vi "XBox-Init.vi"(11 "error in (no error)":errorcluster) -> (4 "XBox Events":T2, 14 "Events Ref":T1, 15 "error out":errorcluster)   [LabVIEW 2015]
uses:
  XBox-Button Event.ctl
  XBox-Events Ref.ctl
  XBox-Globals.vi
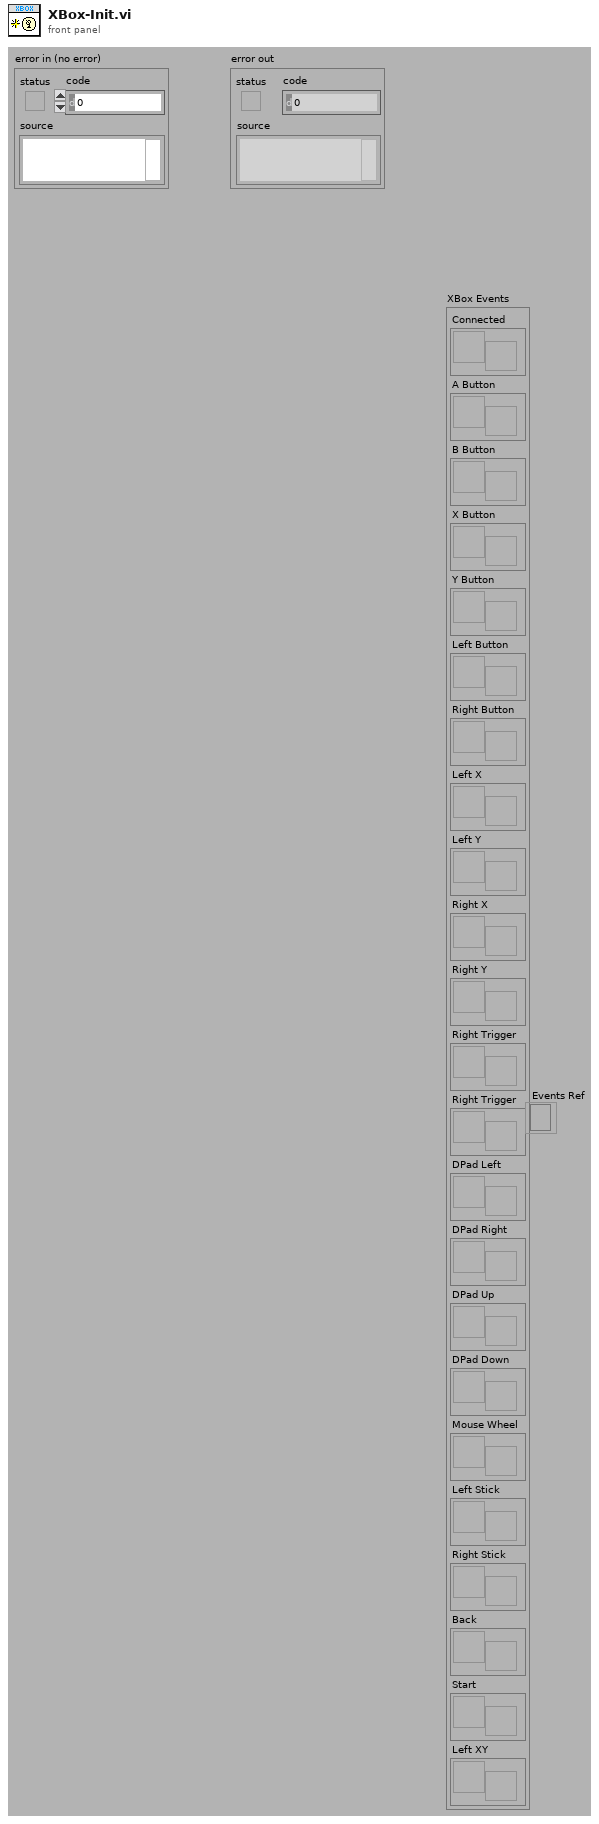
[diagram p1: front panel]
types:
  T1 = typedef "XBox-Events Ref.ctl" = refnum<event-registration>
  T2 = cluster{"Connected":refnum<user-event>, "A Button":refnum<user-event>, "B Button":refnum<user-event>, "X Button":refnum<user-event>, "Y Button":refnum<user-event>, "Left Button":refnum<user-event>, "Right Button":refnum<user-event>, "Left X":refnum<user-event>, "Left Y":refnum<user-event>, "Right X":refnum<user-event>, "Right Y":refnum<user-event>, "Right Trigger":refnum<user-event>, "Right Trigger":refnum<user-event>, "DPad Left":refnum<user-event>, "DPad Right":refnum<user-event>, "DPad Up":refnum<user-event>, "DPad Down":refnum<user-event>, "Mouse Wheel":refnum<user-event>, "Left Stick":refnum<user-event>, "Right Stick":refnum<user-event>, "Back":refnum<user-event>, "Start":refnum<user-event>, "Left XY":refnum<user-event>}
  T3 = typedef "XBox-Button Event.ctl" = cluster{"Down":bool, "Pressed":bool, "Released":bool}
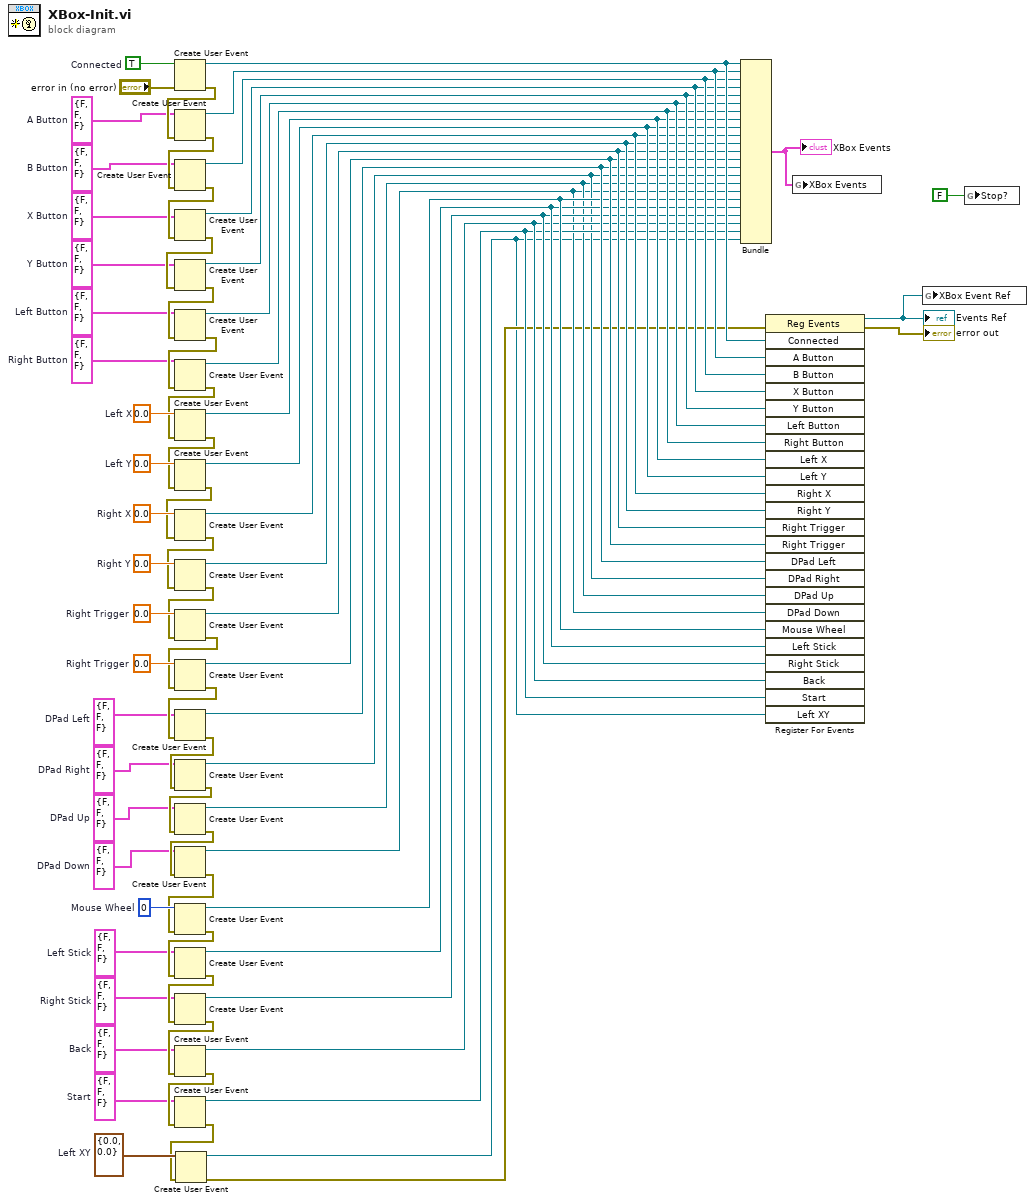
[diagram p0: block diagram]
diagram:
  w5 = cluster{"X":dbl, "Y":dbl} {"X"=0.0, "Y"=0.0}  # Left XY
  w10 = T3 {"Down"=FALSE, "Pressed"=FALSE, "Released"=FALSE}  # DPad Down
  w11 = T3 {"Down"=FALSE, "Pressed"=FALSE, "Released"=FALSE}  # DPad Up
  w12 = T3 {"Down"=FALSE, "Pressed"=FALSE, "Released"=FALSE}  # DPad Right
  w13 = T3 {"Down"=FALSE, "Pressed"=FALSE, "Released"=FALSE}  # DPad Left
  w18 = T3 {"Down"=FALSE, "Pressed"=FALSE, "Released"=FALSE}  # Start
  w19 = T3 {"Down"=FALSE, "Pressed"=FALSE, "Released"=FALSE}  # Back
  w20 = T3 {"Down"=FALSE, "Pressed"=FALSE, "Released"=FALSE}  # Right Stick
  w21 = T3 {"Down"=FALSE, "Pressed"=FALSE, "Released"=FALSE}  # Left Stick
  w22 = T3 {"Down"=FALSE, "Pressed"=FALSE, "Released"=FALSE}  # Right Button
  w23 = T3 {"Down"=FALSE, "Pressed"=FALSE, "Released"=FALSE}  # Left Button
  w24 = T3 {"Down"=FALSE, "Pressed"=FALSE, "Released"=FALSE}  # Y Button
  w25 = T3 {"Down"=FALSE, "Pressed"=FALSE, "Released"=FALSE}  # X Button
  w26 = T3 {"Down"=FALSE, "Pressed"=FALSE, "Released"=FALSE}  # B Button
  w27 = T3 {"Down"=FALSE, "Pressed"=FALSE, "Released"=FALSE}  # A Button
  w67 = TRUE  # Connected
  w68 = 0  # Mouse Wheel
  w69 = 0.0  # Right Trigger
  w70 = 0.0  # Right Trigger
  w71 = 0.0  # Right Y
  w72 = 0.0  # Right X
  w73 = 0.0  # Left Y
  w74 = 0.0  # Left X
  n1 = Create User Event(user event datatype=w67, error in="error in (no error)") -> (user event=w51:refnum<user-event>, error out=w66:errorcluster)
  n2 = Create User Event(user event datatype=w27, error in=w66) -> (user event=w50:refnum<user-event>, error out=w65:errorcluster)
  n3 = Create User Event(user event datatype=w26, error in=w65) -> (user event=w49:refnum<user-event>, error out=w64:errorcluster)
  n4 = Create User Event(user event datatype=w25, error in=w64) -> (user event=w48:refnum<user-event>, error out=w63:errorcluster)
  n5 = Create User Event(user event datatype=w24, error in=w63) -> (user event=w47:refnum<user-event>, error out=w62:errorcluster)
  n6 = Create User Event(user event datatype=w23, error in=w62) -> (user event=w46:refnum<user-event>, error out=w61:errorcluster)
  n7 = Create User Event(user event datatype=w22, error in=w61) -> (user event=w45:refnum<user-event>, error out=w60:errorcluster)
  n8 = Create User Event(user event datatype=w74, error in=w60) -> (user event=w44:refnum<user-event>, error out=w59:errorcluster)
  n9 = Create User Event(user event datatype=w73, error in=w59) -> (user event=w43:refnum<user-event>, error out=w58:errorcluster)
  n10 = Create User Event(user event datatype=w72, error in=w58) -> (user event=w42:refnum<user-event>, error out=w57:errorcluster)
  n11 = Create User Event(user event datatype=w71, error in=w57) -> (user event=w41:refnum<user-event>, error out=w56:errorcluster)
  n12 = Create User Event(user event datatype=w70, error in=w56) -> (user event=w40:refnum<user-event>, error out=w55:errorcluster)
  n13 = Create User Event(user event datatype=w69, error in=w55) -> (user event=w39:refnum<user-event>, error out=w54:errorcluster)
  n14 = Create User Event(user event datatype=w13, error in=w54) -> (user event=w38:refnum<user-event>, error out=w17:errorcluster)
  n15 = Create User Event(user event datatype=w12, error in=w17) -> (user event=w8:refnum<user-event>, error out=w16:errorcluster)
  n16 = Create User Event(user event datatype=w11, error in=w16) -> (user event=w7:refnum<user-event>, error out=w15:errorcluster)
  n17 = Create User Event(user event datatype=w10, error in=w15) -> (user event=w6:refnum<user-event>, error out=w14:errorcluster)
  n18 = Create User Event(user event datatype=w68, error in=w14) -> (user event=w37:refnum<user-event>, error out=w31:errorcluster)
  n19 = Create User Event(user event datatype=w21, error in=w31) -> (user event=w35:refnum<user-event>, error out=w30:errorcluster)
  n20 = Create User Event(user event datatype=w20, error in=w30) -> (user event=w34:refnum<user-event>, error out=w29:errorcluster)
  n21 = Create User Event(user event datatype=w19, error in=w29) -> (user event=w33:refnum<user-event>, error out=w28:errorcluster)
  n22 = Create User Event(user event datatype=w18, error in=w28) -> (user event=w32:refnum<user-event>, error out=w4:errorcluster)
  n23 = Create User Event(user event datatype=w5, error in=w4) -> (user event=w2:refnum<user-event>, error out=w3:errorcluster)
  n24 = Bundle("Connected"=w51, "A Button"=w50, "B Button"=w49, "X Button"=w48, "Y Button"=w47, "Left Button"=w46, "Right Button"=w45, "Left X"=w44, "Left Y"=w43, "Right X"=w42, "Right Y"=w41, "Right Trigger"=w40, "Right Trigger"=w39, "DPad Left"=w38, "DPad Right"=w8, "DPad Up"=w7, "DPad Down"=w6, "Mouse Wheel"=w37, "Left Stick"=w35, "Right Stick"=w34, "Back"=w33, "Start"=w32, "Left XY"=w2) -> (w9:T2)  [unwired: 1 in]
  "XBox Events" <- w9
  n25 = register-events(error in=w3, w51, w50, w49, w48, w47, w46, w45, w44, w43, w42, w41, w40, w39, w38, w8, w7, w6, w37, w35, w34, w33, w32, w2) -> (reference out=w1:refnum<event-registration>, error out=→"error out":errorcluster)  [unwired: 1 in]
  "Events Ref" <- w1
  n26 = global write "XBox-Globals.vi" "XBox Events"(w9) -> ()
  n27 = global write "XBox-Globals.vi" "XBox Event Ref"(w1) -> ()
  n28 = global write "XBox-Globals.vi" "Stop?"(FALSE ("Stop?")) -> ()
